vi "Autonomous Independent.vi"() -> ()   [LabVIEW 2014]
doc: "This VI is called when autonomous begins, and will automatically be terminated when autonomous ends. You can carry out timed or sensor driven robot movement independently without needing to return to the caller."
uses:
  <vilib>/Rock Robotics/WPI/Solenoid/WPI_SolenoidValue.ctl
  <vilib>/Rock Robotics/WPI/SafetyOutput/WPI_SafetyOutputConfigMenu.ctl
  <vilib>/Rock Robotics/WPI/RobotDrive/WPI_RobotDriveGetSetRefNum.vi
  <vilib>/Rock Robotics/Network Tables/SD Read Numeric Array.vi
  <vilib>/Rock Robotics/WPI/Solenoid/WPI_SolenoidSetEnum.vi
  Robot Global Data.vi
panel:
  in  "Intake Wheels deployed?":bool=TRUE
  in  "Tote Count":dbl
  in  "Internal Tote Slot open?":bool
  in  "Object in Arm?":bool
  # "Be sure to right-click and choose Data Operations>>Make Current Value default if you want to save the array values with the VI"
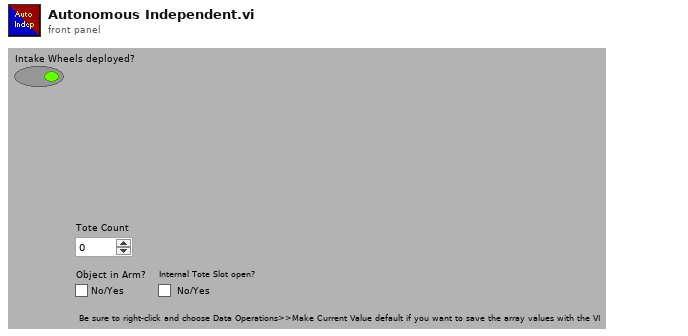
[diagram p1: front panel]
types:
  T1 = typedef "WPI_MotorControlDeviceRef.ctl" = cluster{"DeviceStatus":errorcluster, "Type":T2, "PWM":cluster{"Controller":T3, "PWM Channel":T4, "DeadBand":T5}, "CAN":cluster{"Device Number":u8, "Control Mode":T6, "Semaphore":T7, "Max Vout":dbl, "TalonSRX Control Mode":T8}, "Invert":bool, "TransformRef":T9, "InvTransformRef":T9}
  T2 = typedef "WPI_MotorControlType.ctl" = enum16{"PWM", "CAN", "CANTalonSRX"}
  T3 = typedef "FPGA_TypedefDigitalModule.ctl" = enum16{"Controller 1"}
  T4 = typedef "FPGA_DIOPWMChannel.ctl" = enum8{"PWM 0", "PWM 1", "PWM 2", "PWM 3", "PWM 4", "PWM 5", "PWM 6", "PWM 7", "PWM 8", "PWM 9", "PWM MXP 0", "PWM MXP 1", "PWM MXP 2", "PWM MXP 3", "PWM MXP 4", "PWM MXP 5", "PWM MXP 6", "PWM MXP 7", "PWM MXP 8", "PWM MXP 9", "Invalid"}
  T5 = typedef "WPI_PWMDeadband.ctl" = cluster{"Name":string, "maxPositivePwm":i32, "minPositivePwm":i32, "centerPwm":i32, "maxNegativePwm":i32, "minNegativePwm":i32, "angularRange":u16}
  T6 = typedef "WPI_CANJaguar_ControlMode.ctl" = enum8{"Percent VBus", "Current", "Speed", "Position", "Voltage"}
  T7 = typedef "Semaphore RefNum" = refnum<k1>
  T8 = typedef "WPI_CANTalonSRX_APIControlMode.ctl" = enum8{"Percent VBus", "Speed", "Position", "Slave", "Unchanged / Invalid"}
  T9 = typedef "WPI_PWMTransform_ConPane.ctl" = refnum<vi>
  T10 = typedef "WPI_RobotDriveDevRef.ctl" = cluster{"DevStatus":errorcluster, "Motors[]":T1[], "Square Inputs":bool, "Max Output":dbl}
  T11 = typedef "WPI_SolenoidDevRef.ctl" = cluster{"DevStatus":errorcluster, "Pneumatics Control Module":u8, "Forward Solenoid Channel":T12, "Reverse Solenoid Channel":T12}
  T12 = typedef "WPI_SolenoidChannel.ctl" = enum8{"Solenoid 0", "Solenoid 1", "Solenoid 2", "Solenoid 3", "Solenoid 4", "Solenoid 5", "Solenoid 6", "Solenoid 7", "Invalid"}
  T13 = typedef "WPI_SafetyOutputConfigMenu.ctl" = enum16{"Enable", "Disable"}
  T14 = typedef "WPI_SolenoidValue.ctl" = enum16{"Off", "On", "Forward", "Reverse"}
  T15 = cluster{"Numeric Array[0]":dbl, "Numeric Array[1]":dbl, "Numeric Array[2]":dbl, "Numeric Array[3]":dbl, "Numeric Array[4]":dbl, "Numeric Array[5]":dbl, "Numeric Array[6]":dbl, "Numeric Array[7]":dbl, "Numeric Array[8]":dbl}
  T16 = cluster{"Numeric Array[0]":dbl, "Numeric Array[1]":dbl, "Numeric Array[2]":dbl}
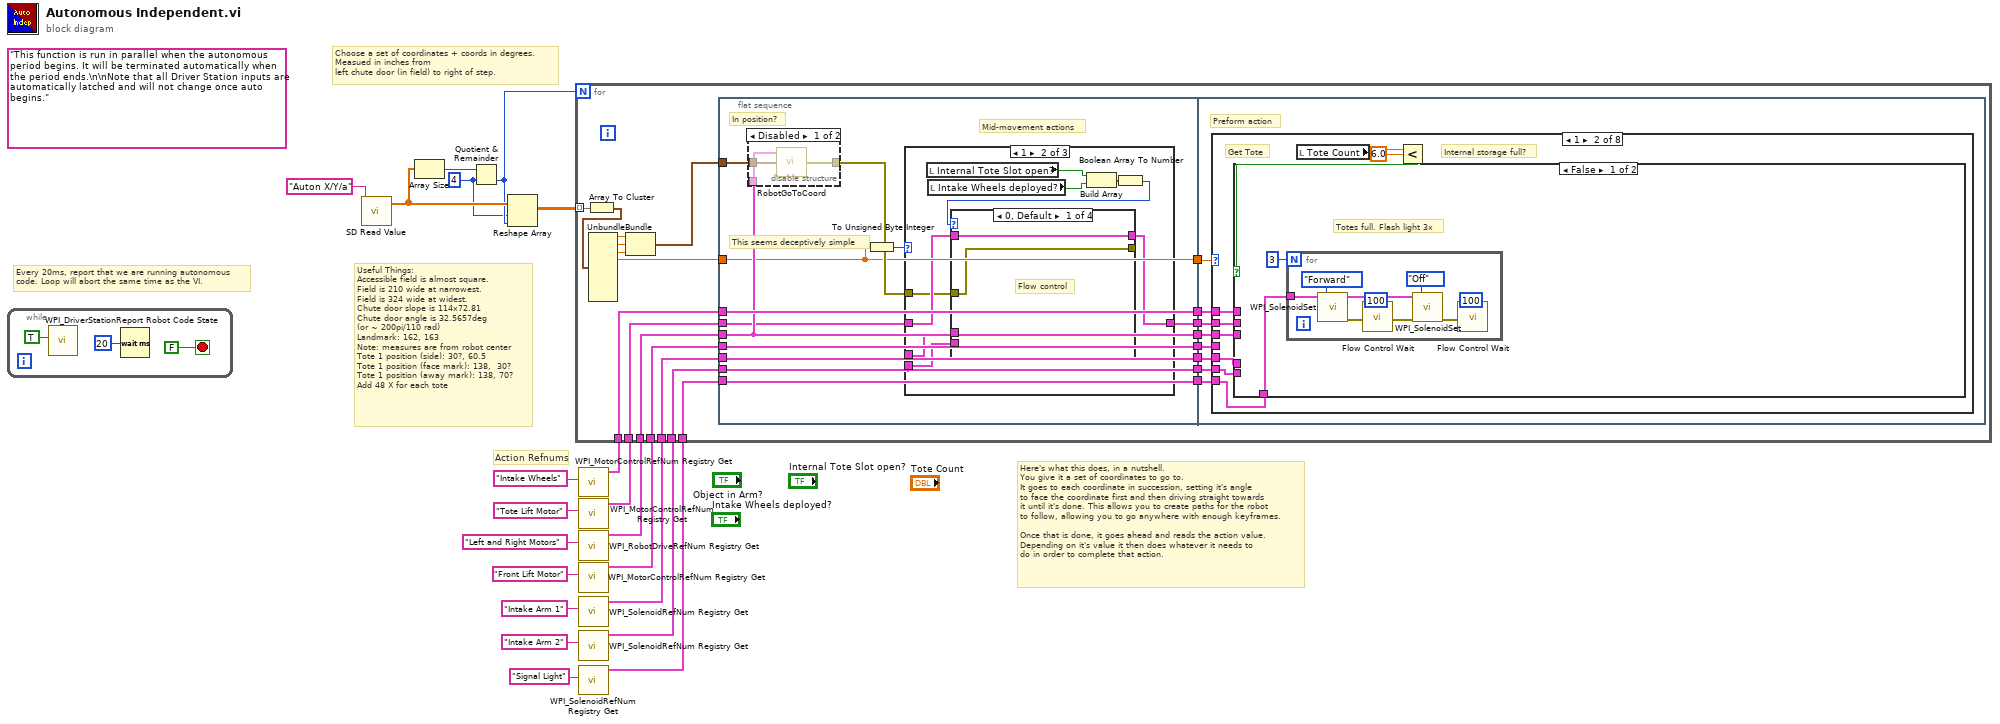
[diagram p0: block diagram]
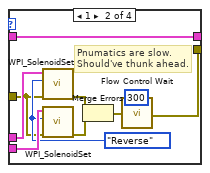
[diagram p4: hidden frame]
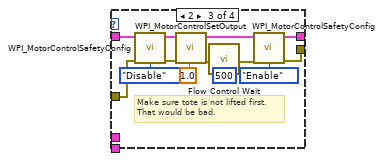
[diagram p5: hidden frame]
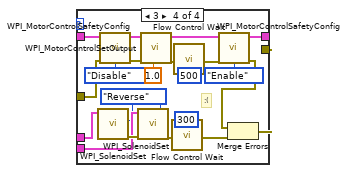
[diagram p6: hidden frame]
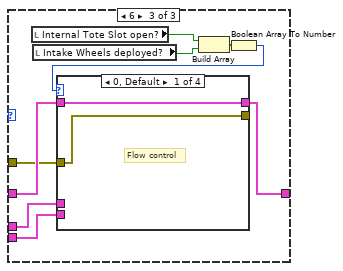
[diagram p7: hidden frame]
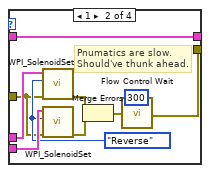
[diagram p8: hidden frame]
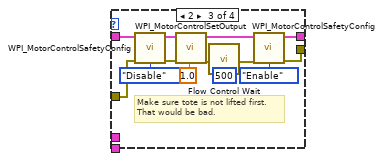
[diagram p9: hidden frame]
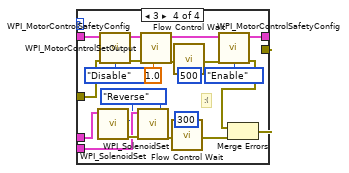
[diagram p10: hidden frame]
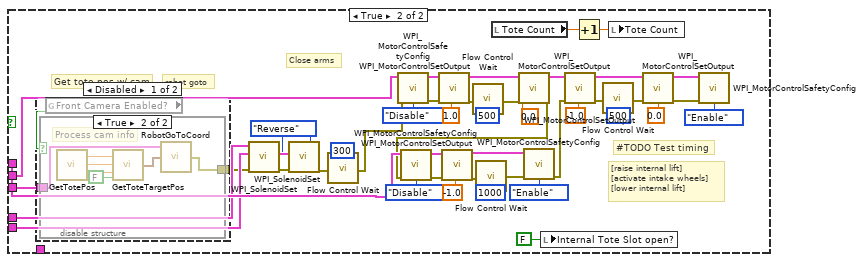
[diagram p12: hidden frame]
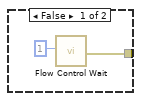
[diagram p13: hidden frame]
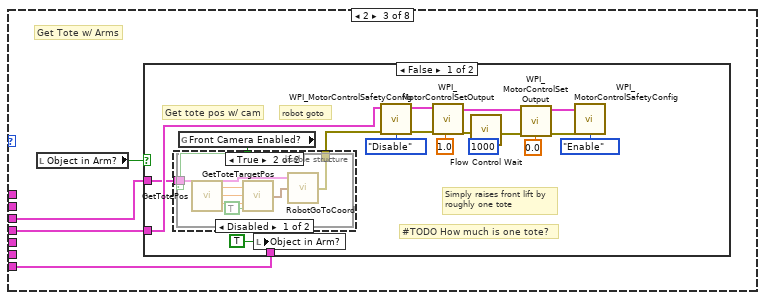
[diagram p15: hidden frame]
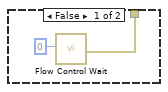
[diagram p16: hidden frame]
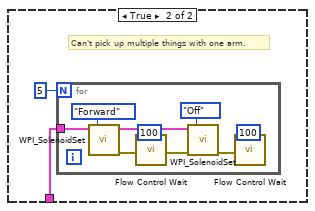
[diagram p18: hidden frame]
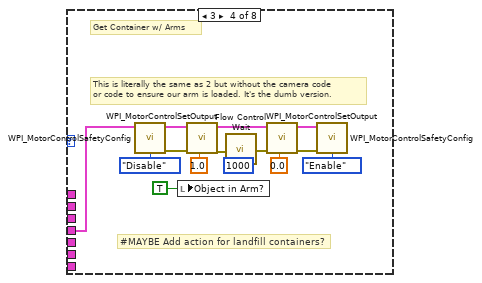
[diagram p19: hidden frame]
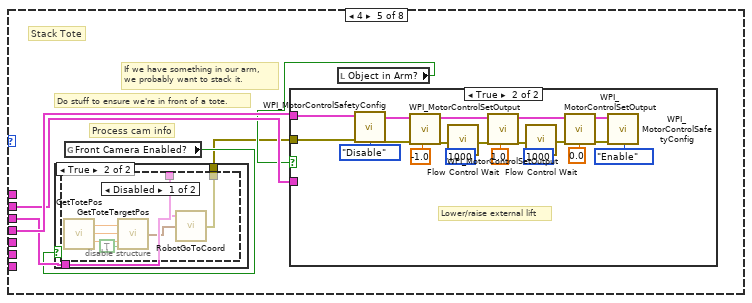
[diagram p20: hidden frame]
diagram:
  w16 = 4 ("y")
  (unwired) "This function is run in parallel when the autonomous period begins. It will be terminated automatically when the period ends.\n\nNote that all Driver Station inputs are automatically latched and will not change once auto begins."
  # "Action Refnums"
  # "Useful Things:\nAccessible field is almost square.\nField is 210 wide at narrowest.\nField is 324 wide at widest. \nChute door slope is 114x72.81\nChute door angle is 32.5657deg\n(or ~ 200pi/110 rad) \nLandmark: 162, 163\nNote: measures are from robot center\nTote 1 position (side): 30?, 60.5 \nTote 1 position (face mark): 138,  30?\nTote 1 position (away mark): 138, 70? \nAdd 48 X for each tote"
  # "Choose a set of coordinates + coords in degrees.\nMeasued in inches from\nleft chute door (in field) to right of step."
  # "Here's what this does, in a nutshell.\nYou give it a set of coordinates to go to.\nIt goes to each coordinate in succession, setting it's angle\nto face the coordinate first and then driving straight towards\nit until it's done. This allows you to create paths for the robot\nto follow, allowing you to go anywhere with enough keyframes.\n\nOnce that is done, it goes ahead and reads the action value.\nDepending on it's value it then does whatever it needs to\ndo in order to complete that action."
  # "Every 20ms, report that we are running autonomous\ncode. Loop will abort the same time as the VI."
  n1 = while {
    stop <- FALSE stop-if-true
    n2 = call <vilib>:"WPI_DriverStationReport Robot Code State.vi"("Autonomous"=TRUE) -> ()  [unwired: 10 in, 1 out]
    n3 = Wait (ms)(milliseconds to wait=u32 20) -> ()  [unwired: 1 out]
  }
  n4 = call-poly <vilib>:"SD Read Value.vi"("Name"="Auton X/Y/a") -> ("Numeric Array"=w19:dbl[])  [unwired: 8 in, 2 out]
  n5 = Array Size(array=w19) -> (size(s)=w20:i32)
  n6 = Quotient & Remainder(x=w20, y=w16) -> (floor(x/y)=w17:i32)  [unwired: 1 out]
  n7 = Reshape Array(w19, w16, w17) -> (w18:dbl[][])
  n8 = call <vilib>:"WPI_MotorControlRefNum Registry Get.vi"("refnum name"="Intake Wheels") -> ("MotorControlDevRef"=w14:T1)  [unwired: 9 in, 1 out]
  n9 = call <vilib>:"WPI_MotorControlRefNum Registry Get.vi"("refnum name"="Tote Lift Motor") -> ("MotorControlDevRef"=w12:T1)  [unwired: 9 in, 1 out]
  n10 = call <vilib>:"WPI_RobotDriveRefNum Registry Get.vi"("refnum name"="Left and Right Motors") -> ("RobotDriveDevRef"=w10:T10)  [unwired: 9 in, 1 out]
  n11 = call <vilib>:"WPI_MotorControlRefNum Registry Get.vi"("refnum name"="Front Lift Motor") -> ("MotorControlDevRef"=w7:T1)  [unwired: 9 in, 1 out]
  n12 = call <vilib>:"WPI_SolenoidRefNum Registry Get.vi"("refnum name"="Intake Arm 1") -> ("SolenoidDevRef"=w4:T11)  [unwired: 9 in, 1 out]
  n13 = call <vilib>:"WPI_SolenoidRefNum Registry Get.vi"("refnum name"="Intake Arm 2") -> ("SolenoidDevRef"=w3:T11)  [unwired: 9 in, 1 out]
  n14 = call <vilib>:"WPI_SolenoidRefNum Registry Get.vi"("refnum name"="Signal Light") -> ("SolenoidDevRef"=w1:T11)  [unwired: 9 in, 1 out]
  n15 = for {
    N: w17 -> [_]
    tunnel: w18 -> [w45] mode=indexing
    tunnel: w14 -> [w38]
    tunnel: w12 -> [w37]
    tunnel: w10 -> [w36]
    tunnel: w7 -> [w35]
    tunnel: w4 -> [w34]
    tunnel: w3 -> [w33]
    tunnel: w1 -> [w25]
    n16 = Array To Cluster(array=w45) -> (cluster=w44:T15)
    n17 = Unbundle(w44) -> ("Numeric Array[0]"=w43:dbl, "Numeric Array[1]"=w42:dbl, "Numeric Array[2]"=w41:dbl, "Numeric Array[3]"=w39:dbl)  [unwired: 5 out]
    n18 = Bundle("Numeric Array[0]"=w43, "Numeric Array[1]"=w42, "Numeric Array[2]"=w41) -> (w40:T16)  [unwired: 1 in]
    n19 = flat-sequence {
      tunnel: w40 -> [w57]
      tunnel: w39 -> [w46]
      tunnel: [w46] -> w32
      tunnel: w38 -> [w56]
      tunnel: [w56] -> w31
      tunnel: w37 -> [w50]
      tunnel: w36 -> [w54]
      tunnel: [w54] -> w30
      tunnel: w35 -> [w55]
      tunnel: [w55] -> w29
      tunnel: w34 -> [w53]
      tunnel: [w53] -> w28
      tunnel: w33 -> [w52]
      tunnel: [w52] -> w27
      tunnel: [w51] -> w26
      tunnel: w25 -> [w49]
      tunnel: [w49] -> w24
      tunnel: w32 -> [w179]
      tunnel: w31 -> [w178]
      tunnel: w30 -> [w176]
      tunnel: w29 -> [w175]
      tunnel: w28 -> [w174]
      tunnel: w27 -> [w173]
      tunnel: w26 -> [w177]
      tunnel: w24 -> [w172]
      frame #0 {
        # "Mid-movement actions"
        # "This seems deceptively simple"
        # "In position?"
        n20 = disable-structure shown="Disabled" {
          disable-tunnel: w57 -> [w60 _]
          disable-tunnel: w54 -> [w59 _]
          disable-tunnel: [w58 _] -> w48
          frame Disabled {
            n21 = call "RobotGoToCoord.vi"("X/Y/a Target"=w60, "RobotDriveDevRef"=w59) -> ("error out"=w58:errorcluster)  [unwired: 1 in]
          }
          frame Enabled {
          }
        }
        n22 = To Unsigned Byte Integer(number=w46) -> (unsigned 8bit integer=w47:u8)
        n23 = case shown="1" w47 {
          tunnel: w50 -> [w61 w67 w122]
          tunnel: w53 -> [_ w66 w121]
          tunnel: w52 -> [_ w65 w120]
          tunnel: [w61 w64 w119] -> w51
          tunnel: w48 -> [_ w62 w117]
          frame 0, Default {
            # "Passthrough so mid-movement actions\ncomplete before post-movement actions"
            # "Do nothing"
          }
          frame 1 {
            n24 = local read "Internal Tote Slot open?"() -> (w70:bool)
            n25 = local read "Intake Wheels deployed?"() -> (w69:bool)
            n26 = Build Array(w70, w69) -> (w63:bool[])
            n27 = Boolean Array To Number(Boolean array=w63) -> (number=w68:u32)
            n28 = case shown="0, Default" w68 {
              tunnel: w67 -> [w72 w74 w86 w102]
              tunnel: [w71 w75 w85 w100] -> _
              tunnel: w66 -> [_ w82 _ w113]
              tunnel: w65 -> [_ w81 _ w112]
              tunnel: [w72 w74 w84 w97] -> w64
              tunnel: w62 -> [w71 w73 w83 w96]
              frame 0, Default {
                # "Flow control"
              }
              frame 1 {
                w80 = WPI_SolenoidValue."Reverse" ("Value")
                # "Pnumatics are slow.\nShould've thunk ahead."
                n29 = call-poly <vilib>:"WPI_SolenoidSet.vi"("error in (no error)"=w73, "Value"=w80, "SolenoidDevRef"=w82) -> ("error out"=w79:errorcluster)  [unwired: 7 in, 1 out]
                n30 = call-poly <vilib>:"WPI_SolenoidSet.vi"("error in (no error)"=w73, "Value"=w80, "SolenoidDevRef"=w81) -> ("error out"=w78:errorcluster)  [unwired: 7 in, 1 out]
                n31 = Merge Errors(w79, w78) -> (w77:errorcluster)
                n32 = call "Flow Control Wait.vi"("milliseconds to wait"=u32 300, "error in (no error)"=w77) -> ("error out"=w75:errorcluster)  [unwired: 17 in]
              }
              frame 2 {
                # "Make sure tote is not lifted first.\nThat would be bad."
                n33 = call <vilib>:"WPI_MotorControlSafetyConfig.vi"("error in (no error)"=w83, "mode"=WPI_SafetyOutputConfigMenu."Disable", "MotorControlDevRef"=w86) -> ("error out"=w93:errorcluster, "MotorControlDevRef"=w94:T1)  [unwired: 7 in]
                n34 = call <vilib>:"WPI_MotorControlSetOutput.vi"("error in (no error)"=w93, "Output"=1.0, "MotorControlDevRef"=w94) -> ("error out"=w92:errorcluster, "MotorControlDevRef"=w89:T1)  [unwired: 6 in, 1 out]
                n35 = call "Flow Control Wait.vi"("milliseconds to wait"=u32 500, "error in (no error)"=w92) -> ("error out"=w88:errorcluster)  [unwired: 17 in]
                n36 = call <vilib>:"WPI_MotorControlSafetyConfig.vi"("error in (no error)"=w88, "mode"=WPI_SafetyOutputConfigMenu."Enable", "MotorControlDevRef"=w89) -> ("error out"=w85:errorcluster, "MotorControlDevRef"=w84:T1)  [unwired: 7 in]
              }
              frame 3 {
                w99 = WPI_SolenoidValue."Reverse" ("Value")
                # ":("
                n37 = call-poly <vilib>:"WPI_SolenoidSet.vi"("Value"=w99, "SolenoidDevRef"=w113) -> ("error out"=w114:errorcluster)  [unwired: 8 in, 1 out]
                n38 = call <vilib>:"WPI_MotorControlSafetyConfig.vi"("error in (no error)"=w96, "mode"=WPI_SafetyOutputConfigMenu."Disable", "MotorControlDevRef"=w102) -> ("error out"=w109:errorcluster, "MotorControlDevRef"=w110:T1)  [unwired: 7 in]
                n39 = call-poly <vilib>:"WPI_SolenoidSet.vi"("error in (no error)"=w114, "Value"=w99, "SolenoidDevRef"=w112) -> ("error out"=w115:errorcluster)  [unwired: 7 in, 1 out]
                n40 = call <vilib>:"WPI_MotorControlSetOutput.vi"("error in (no error)"=w109, "Output"=1.0, "MotorControlDevRef"=w110) -> ("error out"=w108:errorcluster, "MotorControlDevRef"=w105:T1)  [unwired: 6 in, 1 out]
                n41 = call "Flow Control Wait.vi"("milliseconds to wait"=u32 300, "error in (no error)"=w115) -> ("error out"=w101:errorcluster)  [unwired: 17 in]
                n42 = call "Flow Control Wait.vi"("milliseconds to wait"=u32 500, "error in (no error)"=w108) -> ("error out"=w104:errorcluster)  [unwired: 17 in]
                n43 = call <vilib>:"WPI_MotorControlSafetyConfig.vi"("error in (no error)"=w104, "mode"=WPI_SafetyOutputConfigMenu."Enable", "MotorControlDevRef"=w105) -> ("error out"=w98:errorcluster, "MotorControlDevRef"=w97:T1)  [unwired: 7 in]
                n44 = Merge Errors(w98, w101) -> (w100:errorcluster)
              }
            }
          }
          frame 6 {
            n45 = local read "Internal Tote Slot open?"() -> (w125:bool)
            n46 = local read "Intake Wheels deployed?"() -> (w124:bool)
            n47 = Build Array(w125, w124) -> (w118:bool[])
            n48 = Boolean Array To Number(Boolean array=w118) -> (number=w123:u32)
            n49 = case shown="0, Default" w123 {
              tunnel: w122 -> [w127 w129 w141 w157]
              tunnel: [w126 w130 w140 w155] -> _
              tunnel: w121 -> [_ w137 _ w168]
              tunnel: w120 -> [_ w136 _ w167]
              tunnel: [w127 w129 w139 w152] -> w119
              tunnel: w117 -> [w126 w128 w138 w151]
              frame 0, Default {
                # "Flow control"
              }
              frame 1 {
                w135 = WPI_SolenoidValue."Reverse" ("Value")
                # "Pnumatics are slow.\nShould've thunk ahead."
                n50 = call-poly <vilib>:"WPI_SolenoidSet.vi"("error in (no error)"=w128, "Value"=w135, "SolenoidDevRef"=w137) -> ("error out"=w134:errorcluster)  [unwired: 7 in, 1 out]
                n51 = call-poly <vilib>:"WPI_SolenoidSet.vi"("error in (no error)"=w128, "Value"=w135, "SolenoidDevRef"=w136) -> ("error out"=w133:errorcluster)  [unwired: 7 in, 1 out]
                n52 = Merge Errors(w134, w133) -> (w132:errorcluster)
                n53 = call "Flow Control Wait.vi"("milliseconds to wait"=u32 300, "error in (no error)"=w132) -> ("error out"=w130:errorcluster)  [unwired: 17 in]
              }
              frame 2 {
                # "Make sure tote is not lifted first.\nThat would be bad."
                n54 = call <vilib>:"WPI_MotorControlSafetyConfig.vi"("error in (no error)"=w138, "mode"=WPI_SafetyOutputConfigMenu."Disable", "MotorControlDevRef"=w141) -> ("error out"=w148:errorcluster, "MotorControlDevRef"=w149:T1)  [unwired: 7 in]
                n55 = call <vilib>:"WPI_MotorControlSetOutput.vi"("error in (no error)"=w148, "Output"=1.0, "MotorControlDevRef"=w149) -> ("error out"=w147:errorcluster, "MotorControlDevRef"=w144:T1)  [unwired: 6 in, 1 out]
                n56 = call "Flow Control Wait.vi"("milliseconds to wait"=u32 500, "error in (no error)"=w147) -> ("error out"=w143:errorcluster)  [unwired: 17 in]
                n57 = call <vilib>:"WPI_MotorControlSafetyConfig.vi"("error in (no error)"=w143, "mode"=WPI_SafetyOutputConfigMenu."Enable", "MotorControlDevRef"=w144) -> ("error out"=w140:errorcluster, "MotorControlDevRef"=w139:T1)  [unwired: 7 in]
              }
              frame 3 {
                w154 = WPI_SolenoidValue."Reverse" ("Value")
                # ":("
                n58 = call-poly <vilib>:"WPI_SolenoidSet.vi"("Value"=w154, "SolenoidDevRef"=w168) -> ("error out"=w169:errorcluster)  [unwired: 8 in, 1 out]
                n59 = call <vilib>:"WPI_MotorControlSafetyConfig.vi"("error in (no error)"=w151, "mode"=WPI_SafetyOutputConfigMenu."Disable", "MotorControlDevRef"=w157) -> ("error out"=w164:errorcluster, "MotorControlDevRef"=w165:T1)  [unwired: 7 in]
                n60 = call-poly <vilib>:"WPI_SolenoidSet.vi"("error in (no error)"=w169, "Value"=w154, "SolenoidDevRef"=w167) -> ("error out"=w170:errorcluster)  [unwired: 7 in, 1 out]
                n61 = call <vilib>:"WPI_MotorControlSetOutput.vi"("error in (no error)"=w164, "Output"=1.0, "MotorControlDevRef"=w165) -> ("error out"=w163:errorcluster, "MotorControlDevRef"=w160:T1)  [unwired: 6 in, 1 out]
                n62 = call "Flow Control Wait.vi"("milliseconds to wait"=u32 300, "error in (no error)"=w170) -> ("error out"=w156:errorcluster)  [unwired: 17 in]
                n63 = call "Flow Control Wait.vi"("milliseconds to wait"=u32 500, "error in (no error)"=w163) -> ("error out"=w159:errorcluster)  [unwired: 17 in]
                n64 = call <vilib>:"WPI_MotorControlSafetyConfig.vi"("error in (no error)"=w159, "mode"=WPI_SafetyOutputConfigMenu."Enable", "MotorControlDevRef"=w160) -> ("error out"=w153:errorcluster, "MotorControlDevRef"=w152:T1)  [unwired: 7 in]
                n65 = Merge Errors(w153, w156) -> (w155:errorcluster)
              }
            }
          }
        }
      }
      frame #1 {
        # "Preform action"
        n66 = case shown="1" w179 {
          tunnel: w178 -> [_ w188 _ _ _ _ w390 _]
          tunnel: w177 -> [_ w184 _ _ w318 _ _ _]
          tunnel: w176 -> [_ w185 w257 _ w317 _ _ _]
          tunnel: w175 -> [_ _ w259 w313 w319 w375 _ _]
          tunnel: w174 -> [_ w187 _ _ _ _ _ _]
          tunnel: w173 -> [_ w186 _ _ _ _ _ _]
          tunnel: w172 -> [_ w180 w256 _ _ _ _ _]
          frame 0, Default {
            # "Do nothing"
          }
          frame 1 {
            # "Internal storage full?"
            # "Get Tote"
            n67 = local read "Tote Count"() -> (w183:dbl)
            n68 = Less?(x=w183, y=6.0) -> (x < y?=w181:bool)
            n69 = case shown="False" w181 {
              tunnel: w188 -> [_ w243]
              tunnel: w187 -> [_ w238]
              tunnel: w186 -> [_ w237]
              tunnel: w185 -> [_ w236]
              tunnel: w184 -> [_ w231]
              tunnel: w180 -> [w189 _]
              frame False {
                # "Totes full. Flash light 3x"
                n70 = for {
                  N: 3 -> [_]
                  tunnel: w189 -> [w198]
                  n71 = call-poly <vilib>:"WPI_SolenoidSet.vi"("Value"=WPI_SolenoidValue."Forward", "SolenoidDevRef"=w198) -> ("error out"=w199:errorcluster, "SolenoidDevRef"=w191:T11)  [unwired: 8 in]
                  n72 = call "Flow Control Wait.vi"("milliseconds to wait"=u32 100, "error in (no error)"=w199) -> ("error out"=w192:errorcluster)  [unwired: 17 in]
                  n73 = call-poly <vilib>:"WPI_SolenoidSet.vi"("error in (no error)"=w192, "Value"=WPI_SolenoidValue."Off", "SolenoidDevRef"=w191) -> ("error out"=w195:errorcluster)  [unwired: 7 in, 1 out]
                  n74 = call "Flow Control Wait.vi"("milliseconds to wait"=u32 100, "error in (no error)"=w195) -> ()  [unwired: 17 in, 1 out]
                }
              }
              frame True {
                w232 = WPI_SolenoidValue."Reverse" ("Value")
                # "[raise internal lift]\n[activate intake wheels]\n[lower internal lift]"
                # "#TODO Test timing"
                # "Close arms"
                # "robot goto"
                # "Get tote pos w/ cam"
                n75 = disable-structure shown="Disabled" {
                  disable-tunnel: w236 -> [w246 _]
                  disable-tunnel: [w244 _] -> w230
                  frame Disabled {
                    n76 = global read "Robot Global Data.vi" "Front Camera Enabled?"() -> (w245:bool)
                    n77 = case shown="True" w245 {
                      tunnel: w246 -> [_ w250]
                      tunnel: [w247 w249] -> w244
                      frame False {
                        n78 = call "Flow Control Wait.vi"("milliseconds to wait"=u32 1) -> ("error out"=w247:errorcluster)  [unwired: 18 in]
                      }
                      frame True {
                        # "Process cam info"
                        n79 = call "GetTotePos.vi"() -> ("X Offset"=w252:dbl, "Angle"=w253:dbl, "Distance"=w254:dbl)  [unwired: 4 in]
                        n80 = call "GetToteTargetPos.vi"("Pick up from Side"=FALSE, "X Offset"=w252, "Angle (rad)"=w253, "Dist"=w254) -> ("Target X/Y/a"=w255:cluster{dbl, dbl, dbl})
                        n81 = call "RobotGoToCoord.vi"("X/Y/a Target"=w255, "RobotDriveDevRef"=w250) -> ("error out"=w249:errorcluster)  [unwired: 1 in]
                      }
                    }
                  }
                  frame Enabled {
                  }
                }
                n82 = call-poly <vilib>:"WPI_SolenoidSet.vi"("error in (no error)"=w230, "Value"=w232, "SolenoidDevRef"=w238) -> ("error out"=w233:errorcluster)  [unwired: 7 in, 1 out]
                n83 = call-poly <vilib>:"WPI_SolenoidSet.vi"("error in (no error)"=w233, "Value"=w232, "SolenoidDevRef"=w237) -> ("error out"=w234:errorcluster)  [unwired: 7 in, 1 out]
                n84 = call "Flow Control Wait.vi"("milliseconds to wait"=u32 300, "error in (no error)"=w234) -> ("error out"=w239:errorcluster)  [unwired: 17 in]
                n85 = call <vilib>:"WPI_MotorControlSafetyConfig.vi"("error in (no error)"=w239, "mode"=WPI_SafetyOutputConfigMenu."Disable", "MotorControlDevRef"=w231) -> ("error out"=w227:errorcluster, "MotorControlDevRef"=w228:T1)  [unwired: 7 in]
                n86 = call <vilib>:"WPI_MotorControlSetOutput.vi"("error in (no error)"=w227, "Output"=1.0, "MotorControlDevRef"=w228) -> ("error out"=w226:errorcluster, "MotorControlDevRef"=w213:T1)  [unwired: 6 in, 1 out]
                n87 = call "Flow Control Wait.vi"("milliseconds to wait"=u32 500, "error in (no error)"=w226) -> ("error out"=w212:errorcluster)  [unwired: 17 in]
                n88 = local read "Tote Count"() -> (w242:dbl)
                n89 = call <vilib>:"WPI_MotorControlSetOutput.vi"("error in (no error)"=w212, "Output"=0.0, "MotorControlDevRef"=w213) -> ("error out"=w208:errorcluster, "MotorControlDevRef"=w204:T1)  [unwired: 6 in, 1 out]
                n90 = call <vilib>:"WPI_MotorControlSafetyConfig.vi"("error in (no error)"=w208, "mode"=WPI_SafetyOutputConfigMenu."Disable", "MotorControlDevRef"=w243) -> ("error out"=w219:errorcluster, "MotorControlDevRef"=w218:T1)  [unwired: 7 in]
                n91 = call <vilib>:"WPI_MotorControlSetOutput.vi"("error in (no error)"=w219, "Output"=-1.0, "MotorControlDevRef"=w218) -> ("error out"=w220:errorcluster, "MotorControlDevRef"=w211:T1)  [unwired: 6 in, 1 out]
                n92 = call "Flow Control Wait.vi"("milliseconds to wait"=u32 1000, "error in (no error)"=w220) -> ("error out"=w210:errorcluster)  [unwired: 17 in]
                n93 = call <vilib>:"WPI_MotorControlSafetyConfig.vi"("error in (no error)"=w210, "mode"=WPI_SafetyOutputConfigMenu."Enable", "MotorControlDevRef"=w211) -> ("error out"=w205:errorcluster)  [unwired: 7 in, 1 out]
                n94 = local write "Internal Tote Slot open?"(FALSE ("Internal Tote Slot open?")) -> ()
                n95 = call <vilib>:"WPI_MotorControlSetOutput.vi"("error in (no error)"=w205, "Output"=-1.0, "MotorControlDevRef"=w204) -> ("error out"=w214:errorcluster, "MotorControlDevRef"=w203:T1)  [unwired: 6 in, 1 out]
                n96 = Increment(x=w242) -> (x+1=w241:dbl)
                n97 = call "Flow Control Wait.vi"("milliseconds to wait"=u32 500, "error in (no error)"=w214) -> ("error out"=w206:errorcluster)  [unwired: 17 in]
                n98 = local write "Tote Count"(w241) -> ()
                n99 = call <vilib>:"WPI_MotorControlSetOutput.vi"("error in (no error)"=w206, "Output"=0.0, "MotorControlDevRef"=w203) -> ("error out"=w201:errorcluster, "MotorControlDevRef"=w202:T1)  [unwired: 6 in, 1 out]
                n100 = call <vilib>:"WPI_MotorControlSafetyConfig.vi"("error in (no error)"=w201, "mode"=WPI_SafetyOutputConfigMenu."Enable", "MotorControlDevRef"=w202) -> ()  [unwired: 7 in, 2 out]
              }
            }
          }
          frame 2 {
            # "Get Tote w/ Arms"
            n101 = local read "Object in Arm?"() -> (w258:bool)
            n102 = case shown="False" w258 {
              tunnel: w259 -> [w276 _]
              tunnel: w257 -> [w274 _]
              tunnel: w256 -> [_ w289]
              frame False {
                # "#TODO How much is one tote?"
                # "Simply raises front lift by\nroughly one tote"
                # "robot goto"
                # "Get tote pos w/ cam"
                n103 = global read "Robot Global Data.vi" "Front Camera Enabled?"() -> (w273:bool)
                n104 = disable-structure shown="Disabled" {
                  disable-tunnel: w274 -> [w279 _]
                  disable-tunnel: w273 -> [w278 _]
                  disable-tunnel: [w277 _] -> w260
                  frame Disabled {
                    n105 = case shown="True" w278 {
                      tunnel: w279 -> [_ w283]
                      tunnel: [w280 w282] -> w277
                      frame False {
                        n106 = call "Flow Control Wait.vi"("milliseconds to wait"=u32 0) -> ("error out"=w280:errorcluster)  [unwired: 18 in]
                      }
                      frame True {
                        n107 = call "GetTotePos.vi"() -> ("X Offset"=w285:dbl, "Angle"=w286:dbl, "Distance"=w287:dbl)  [unwired: 4 in]
                        n108 = call "GetToteTargetPos.vi"("Pick up from Side"=TRUE, "X Offset"=w285, "Angle (rad)"=w286, "Dist"=w287) -> ("Target X/Y/a"=w288:cluster{dbl, dbl, dbl})
                        n109 = call "RobotGoToCoord.vi"("X/Y/a Target"=w288, "RobotDriveDevRef"=w283) -> ("error out"=w282:errorcluster)  [unwired: 1 in]
                      }
                    }
                  }
                  frame Enabled {
                  }
                }
                n110 = local write "Object in Arm?"(TRUE ("Object in Arm?")) -> ()
                n111 = call <vilib>:"WPI_MotorControlSafetyConfig.vi"("error in (no error)"=w260, "mode"=WPI_SafetyOutputConfigMenu."Disable", "MotorControlDevRef"=w276) -> ("error out"=w270:errorcluster, "MotorControlDevRef"=w271:T1)  [unwired: 7 in]
                n112 = call <vilib>:"WPI_MotorControlSetOutput.vi"("error in (no error)"=w270, "Output"=1.0, "MotorControlDevRef"=w271) -> ("error out"=w269:errorcluster, "MotorControlDevRef"=w264:T1)  [unwired: 6 in, 1 out]
                n113 = call "Flow Control Wait.vi"("milliseconds to wait"=u32 1000, "error in (no error)"=w269) -> ("error out"=w263:errorcluster)  [unwired: 17 in]
                n114 = call <vilib>:"WPI_MotorControlSetOutput.vi"("error in (no error)"=w263, "Output"=0.0, "MotorControlDevRef"=w264) -> ("error out"=w262:errorcluster, "MotorControlDevRef"=w265:T1)  [unwired: 6 in, 1 out]
                n115 = call <vilib>:"WPI_MotorControlSafetyConfig.vi"("error in (no error)"=w262, "mode"=WPI_SafetyOutputConfigMenu."Enable", "MotorControlDevRef"=w265) -> ()  [unwired: 7 in, 2 out]
              }
              frame True {
                # "Can't pick up multiple things with one arm."
                n116 = for {
                  N: 5 -> [_]
                  tunnel: w289 -> [w298]
                  n117 = call-poly <vilib>:"WPI_SolenoidSet.vi"("Value"=WPI_SolenoidValue."Forward", "SolenoidDevRef"=w298) -> ("error out"=w299:errorcluster, "SolenoidDevRef"=w291:T11)  [unwired: 8 in]
                  n118 = call "Flow Control Wait.vi"("milliseconds to wait"=u32 100, "error in (no error)"=w299) -> ("error out"=w292:errorcluster)  [unwired: 17 in]
                  n119 = call-poly <vilib>:"WPI_SolenoidSet.vi"("error in (no error)"=w292, "Value"=WPI_SolenoidValue."Off", "SolenoidDevRef"=w291) -> ("error out"=w295:errorcluster)  [unwired: 7 in, 1 out]
                  n120 = call "Flow Control Wait.vi"("milliseconds to wait"=u32 100, "error in (no error)"=w295) -> ()  [unwired: 17 in, 1 out]
                }
              }
            }
          }
          frame 3 {
            # "This is literally the same as 2 but without the camera code\nor code to ensure our arm is loaded. It's the dumb version."
            # "#MAYBE Add action for landfill containers?"
            # "Get Container w/ Arms"
            n121 = call <vilib>:"WPI_MotorControlSafetyConfig.vi"("mode"=WPI_SafetyOutputConfigMenu."Disable", "MotorControlDevRef"=w313) -> ("error out"=w310:errorcluster, "MotorControlDevRef"=w311:T1)  [unwired: 8 in]
            n122 = local write "Object in Arm?"(TRUE ("Object in Arm?")) -> ()
            n123 = call <vilib>:"WPI_MotorControlSetOutput.vi"("error in (no error)"=w310, "Output"=1.0, "MotorControlDevRef"=w311) -> ("error out"=w309:errorcluster, "MotorControlDevRef"=w302:T1)  [unwired: 6 in, 1 out]
            n124 = call "Flow Control Wait.vi"("milliseconds to wait"=u32 1000, "error in (no error)"=w309) -> ("error out"=w303:errorcluster)  [unwired: 17 in]
            n125 = call <vilib>:"WPI_MotorControlSetOutput.vi"("error in (no error)"=w303, "Output"=0.0, "MotorControlDevRef"=w302) -> ("error out"=w300:errorcluster, "MotorControlDevRef"=w301:T1)  [unwired: 6 in, 1 out]
            n126 = call <vilib>:"WPI_MotorControlSafetyConfig.vi"("error in (no error)"=w300, "mode"=WPI_SafetyOutputConfigMenu."Enable", "MotorControlDevRef"=w301) -> ()  [unwired: 7 in, 2 out]
          }
          frame 4 {
            # "If we have something in our arm,\nwe probably want to stack it."
            # "Process cam info"
            # "Do stuff to ensure we're in front of a tote."
            # "Stack Tote"
            n127 = global read "Robot Global Data.vi" "Front Camera Enabled?"() -> (w316:bool)
            n128 = case shown="True" w316 {
              tunnel: w317 -> [_ w323]
              tunnel: [w320 w322] -> w314
              frame False {
                n129 = call "Flow Control Wait.vi"("milliseconds to wait"=u32 0) -> ("error out"=w320:errorcluster)  [unwired: 18 in]
              }
              frame True {
                n130 = disable-structure shown="Disabled" {
                  disable-tunnel: w323 -> [w325 _]
                  disable-tunnel: [w324 _] -> w322
                  frame Disabled {
                    n131 = call "GetTotePos.vi"() -> ("X Offset"=w327:dbl, "Angle"=w328:dbl, "Distance"=w329:dbl)  [unwired: 4 in]
                    n132 = call "GetToteTargetPos.vi"("Pick up from Side"=TRUE, "X Offset"=w327, "Angle (rad)"=w328, "Dist"=w329) -> ("Target X/Y/a"=w330:cluster{dbl, dbl, dbl})
                    n133 = call "RobotGoToCoord.vi"("X/Y/a Target"=w330, "RobotDriveDevRef"=w325) -> ("error out"=w324:errorcluster)  [unwired: 1 in]
                  }
                  frame Enabled {
                  }
                }
              }
            }
            n134 = local read "Object in Arm?"() -> (w315:bool)
            n135 = case shown="True" w315 {
              tunnel: w319 -> [_ w363]
              tunnel: w318 -> [w344 _]
              tunnel: w314 -> [_ w357]
              frame False {
                # "Basically we just lower/lift the tote stack to make room\nfor more totes. Yay!"
                # "Lower/raise internal lift"
                n136 = call <vilib>:"WPI_MotorControlSafetyConfig.vi"("mode"=WPI_SafetyOutputConfigMenu."Disable", "MotorControlDevRef"=w344) -> ("error out"=w333:errorcluster, "MotorControlDevRef"=w334:T1)  [unwired: 8 in]
                n137 = call <vilib>:"WPI_MotorControlSetOutput.vi"("error in (no error)"=w333, "Output"=-1.0, "MotorControlDevRef"=w334) -> ("error out"=w335:errorcluster, "MotorControlDevRef"=w332:T1)  [unwired: 6 in, 1 out]
                n138 = call "Flow Control Wait.vi"("milliseconds to wait"=u32 1000, "error in (no error)"=w335) -> ("error out"=w331:errorcluster)  [unwired: 17 in]
                n139 = call <vilib>:"WPI_MotorControlSetOutput.vi"("error in (no error)"=w331, "Output"=1.0, "MotorControlDevRef"=w332) -> ("error out"=w346:errorcluster, "MotorControlDevRef"=w341:T1)  [unwired: 6 in, 1 out]
                n140 = call "Flow Control Wait.vi"("milliseconds to wait"=u32 1000, "error in (no error)"=w346) -> ("error out"=w342:errorcluster)  [unwired: 17 in]
                n141 = call <vilib>:"WPI_MotorControlSetOutput.vi"("error in (no error)"=w342, "Output"=0.0, "MotorControlDevRef"=w341) -> ("error out"=w339:errorcluster, "MotorControlDevRef"=w340:T1)  [unwired: 6 in, 1 out]
                n142 = local write "Internal Tote Slot open?"(TRUE ("Internal Tote Slot open?")) -> ()
                n143 = call <vilib>:"WPI_MotorControlSafetyConfig.vi"("error in (no error)"=w339, "mode"=WPI_SafetyOutputConfigMenu."Enable", "MotorControlDevRef"=w340) -> ()  [unwired: 7 in, 2 out]
              }
              frame True {
                # "Lower/raise external lift"
                n144 = call <vilib>:"WPI_MotorControlSafetyConfig.vi"("error in (no error)"=w357, "mode"=WPI_SafetyOutputConfigMenu."Disable", "MotorControlDevRef"=w363) -> ("error out"=w351:errorcluster, "MotorControlDevRef"=w352:T1)  [unwired: 7 in]
                n145 = call <vilib>:"WPI_MotorControlSetOutput.vi"("error in (no error)"=w351, "Output"=-1.0, "MotorControlDevRef"=w352) -> ("error out"=w354:errorcluster, "MotorControlDevRef"=w353:T1)  [unwired: 6 in, 1 out]
                n146 = call "Flow Control Wait.vi"("milliseconds to wait"=u32 1000, "error in (no error)"=w354) -> ("error out"=w350:errorcluster)  [unwired: 17 in]
                n147 = call <vilib>:"WPI_MotorControlSetOutput.vi"("error in (no error)"=w350, "Output"=1.0, "MotorControlDevRef"=w353) -> ("error out"=w365:errorcluster, "MotorControlDevRef"=w360:T1)  [unwired: 6 in, 1 out]
                n148 = call "Flow Control Wait.vi"("milliseconds to wait"=u32 1000, "error in (no error)"=w365) -> ("error out"=w362:errorcluster)  [unwired: 17 in]
                n149 = call <vilib>:"WPI_MotorControlSetOutput.vi"("error in (no error)"=w362, "Output"=0.0, "MotorControlDevRef"=w360) -> ("error out"=w359:errorcluster, "MotorControlDevRef"=w361:T1)  [unwired: 6 in, 1 out]
                n150 = call <vilib>:"WPI_MotorControlSafetyConfig.vi"("error in (no error)"=w359, "mode"=WPI_SafetyOutputConfigMenu."Enable", "MotorControlDevRef"=w361) -> ()  [unwired: 7 in, 2 out]
              }
            }
          }
          frame 5 {
            # "It's a very simple command.\nUseful for simple things.\nMake sure you don't turn left into\nyour beautiful object once you've\nput it down, though."
            # "Place Object on Ground"
            n151 = local write "Object in Arm?"(FALSE ("Internal Tote Slot open?")) -> ()
            n152 = call <vilib>:"WPI_MotorControlSafetyConfig.vi"("mode"=WPI_SafetyOutputConfigMenu."Disable", "MotorControlDevRef"=w375) -> ("error out"=w376:errorcluster, "MotorControlDevRef"=w377:T1)  [unwired: 8 in]
            n153 = call <vilib>:"WPI_MotorControlSetOutput.vi"("error in (no error)"=w376, "Output"=-1.0, "MotorControlDevRef"=w377) -> ("error out"=w378:errorcluster, "MotorControlDevRef"=w369:T1)  [unwired: 6 in, 1 out]
            n154 = call "Flow Control Wait.vi"("milliseconds to wait"=u32 1000, "error in (no error)"=w378) -> ("error out"=w373:errorcluster)  [unwired: 17 in]
            n155 = call <vilib>:"WPI_MotorControlSetOutput.vi"("error in (no error)"=w373, "Output"=0.0, "MotorControlDevRef"=w369) -> ("error out"=w371:errorcluster, "MotorControlDevRef"=w370:T1)  [unwired: 6 in, 1 out]
            n156 = call <vilib>:"WPI_MotorControlSafetyConfig.vi"("error in (no error)"=w371, "mode"=WPI_SafetyOutputConfigMenu."Disable", "MotorControlDevRef"=w370) -> ()  [unwired: 7 in, 2 out]
          }
          frame 6 {
            # "Time to go for"
            # "Eject Tote"
            n157 = call <vilib>:"WPI_MotorControlSafetyConfig.vi"("mode"=WPI_SafetyOutputConfigMenu."Disable", "MotorControlDevRef"=w390) -> ("error out"=w383:errorcluster, "MotorControlDevRef"=w396:T1)  [unwired: 8 in]
            n158 = local write "Internal Tote Slot open?"(TRUE ("Internal Tote Slot open?")) -> ()
            n159 = call <vilib>:"WPI_MotorControlSetOutput.vi"("error in (no error)"=w383, "Output"=-1.0, "MotorControlDevRef"=w396) -> ("error out"=w392:errorcluster, "MotorControlDevRef"=w384:T1)  [unwired: 6 in, 1 out]
            n160 = call "Flow Control Wait.vi"("milliseconds to wait"=u32 1500, "error in (no error)"=w392) -> ("error out"=w387:errorcluster)  [unwired: 17 in]
            n161 = call <vilib>:"WPI_MotorControlSetOutput.vi"("error in (no error)"=w387, "Output"=0.0, "MotorControlDevRef"=w384) -> ("error out"=w386:errorcluster, "MotorControlDevRef"=w385:T1)  [unwired: 6 in, 1 out]
            n162 = call <vilib>:"WPI_MotorControlSafetyConfig.vi"("error in (no error)"=w386, "mode"=WPI_SafetyOutputConfigMenu."Enable", "MotorControlDevRef"=w385) -> ()  [unwired: 7 in, 2 out]
          }
          frame 7 {
            # "Keep the same coorinate and keep calling this if you need longer times."
            # "If we're wating for physics or other robots or something"
            # "Wait 1 second"
            n163 = Wait (ms)(milliseconds to wait=u32 1000) -> ()  [unwired: 1 out]
          }
        }
      }
    }
  }
